vi "XML to Variable Cluster.vi"(10 "Name.Sub":string[](array[string]), 11 "After Var Name":string[](array[string])) -> (3 "Variable Clusters out":T1)   [LabVIEW 2015]
uses:
  Variable cluster.ctl
panel:
  out "Array":string[](array[string])
  out "error IO":errorcluster
  in  "error in":errorcluster
  out "Numeric":i32
  in  "Variable Clusters":T1
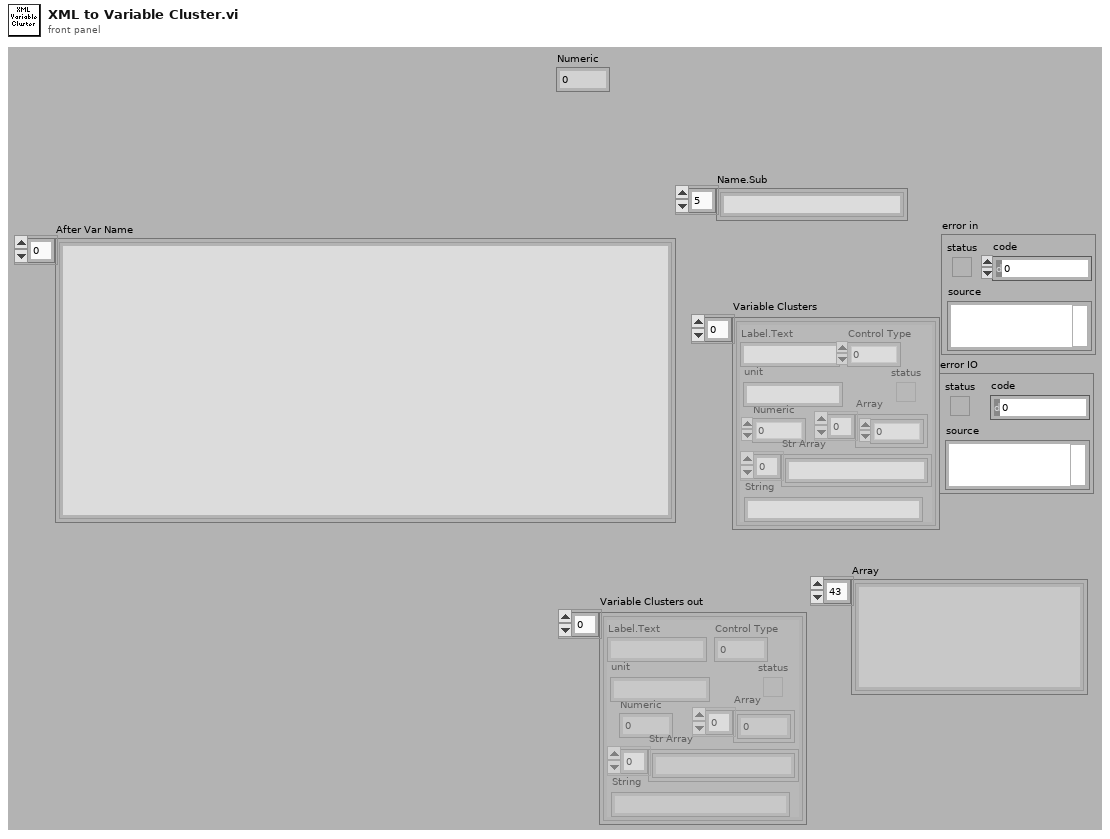
[diagram p1: front panel]
types:
  T1 = typedef "Variable cluster.ctl" = cluster{"Label.Text":string, "Control Type":u32, "Numeric":dbl, "Array":dbl[], "status":bool, "Str Array":string[], "String":string, "unit":string}[]
  T2 = cluster{"Label.Text":string, "Control Type":u32, "Numeric":dbl, "Array":dbl[], "status":bool, "Str Array":string[], "String":string, "unit":string}
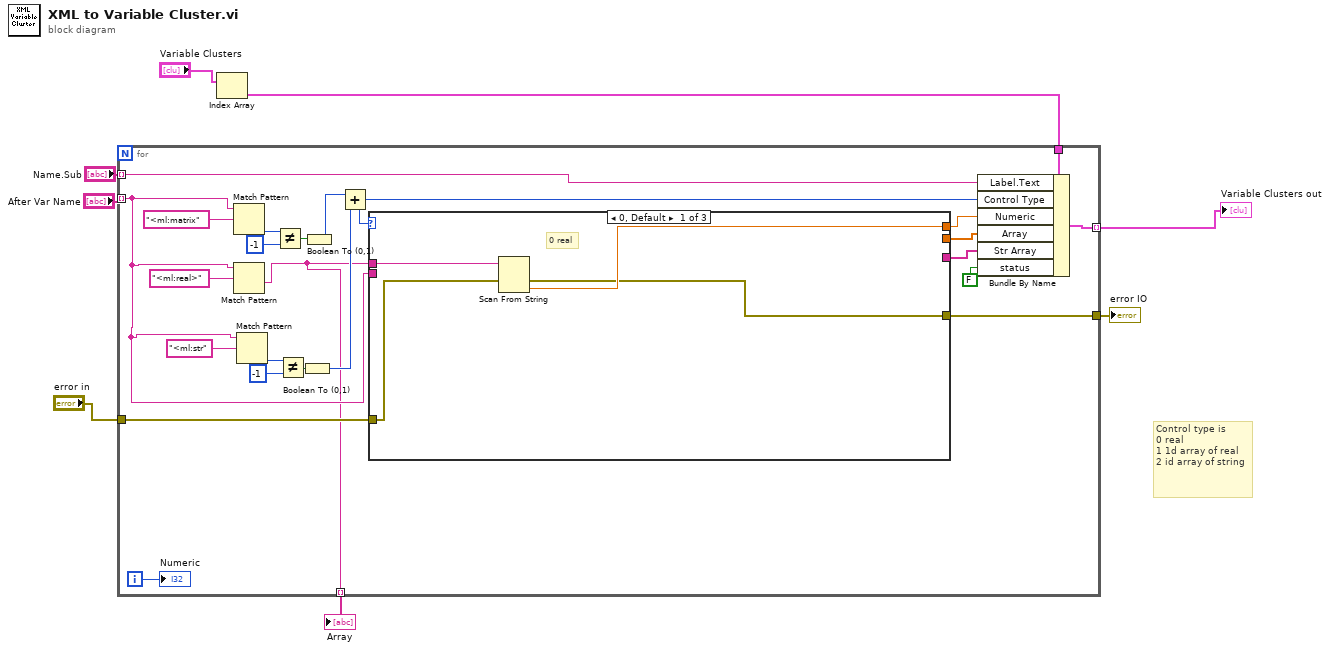
[diagram p0: block diagram]
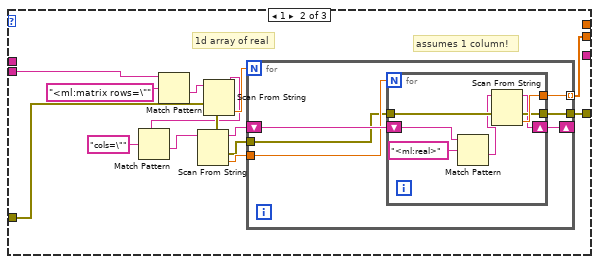
[diagram p2: hidden frame]
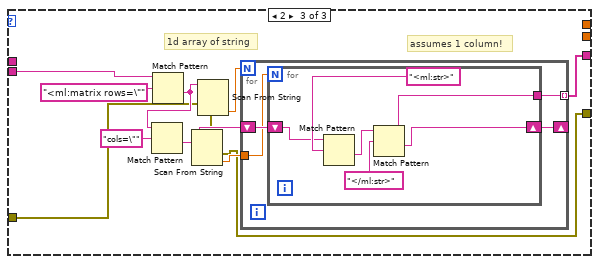
[diagram p3: hidden frame]
diagram:
  # "Control type is\n0 real\n1 1d array of real\n2 id array of string"
  n1 = Index Array(array="Variable Clusters") -> (element=w5:T2)  [unwired: 1 in]
  n2 = for {
    tunnel: "After Var Name" -> [w17] mode=indexing
    tunnel: "Name.Sub" -> [w30] mode=indexing
    tunnel: w5 -> [w32]
    tunnel: [w31] -> w4 mode=indexing
    tunnel: "error in" -> [w12]
    tunnel: [w11] -> w2
    tunnel: [w10] -> w1 mode=indexing
    i -> [w13]
    n3 = Match Pattern(string=w17, regular expression="<ml:matrix") -> (offset past match=w28:i32)  [unwired: 1 in, 3 out]
    n4 = Match Pattern(string=w17, regular expression="<ml:real>") -> (after substring=w10:string)  [unwired: 1 in, 3 out]
    n5 = Match Pattern(string=w17, regular expression="<ml:str") -> (offset past match=w24:i32)  [unwired: 1 in, 3 out]
    n6 = Not Equal?(x=w28, y=-1) -> (x != y?=w22:bool)
    n7 = Not Equal?(x=w24, y=-1) -> (x != y?=w20:bool)
    n8 = Boolean To (0,1)(Boolean=w20) -> (0, 1=w19:i16)
    n9 = Boolean To (0,1)(Boolean=w22) -> (0, 1=w21:i16)
    n10 = Add(x=w21, y=w19) -> (x+y=w18:i16)
    n11 = case shown="0, Default" w18 {
      tunnel: w17 -> [_ w50 w72]
      tunnel: w10 -> [w36 _ _]
      tunnel: [w35 _ _] -> w16
      tunnel: [_ w47 _] -> w15
      tunnel: [_ _ w71] -> w14
      tunnel: w12 -> [w34 w44 w66]
      tunnel: [w33 w41 w64] -> w11
      frame 0, Default {
        # "0 real"
        n12 = Scan From String(input string=w36, error in=w34) -> (error out=w33:errorcluster, output 1=w35:dbl)  [unwired: 3 in, 2 out]
      }
      frame 1 {
        # "assumes 1 column!"
        # "1d array of real"
        n13 = Match Pattern(string=w50, regular expression="<ml:matrix rows=\"") -> (after substring=w40:string)  [unwired: 1 in, 3 out]
        n14 = Scan From String(input string=w40, error in=w44) -> (remaining string=w39:string, error out=w43:errorcluster, output 1=w45:dbl)  [unwired: 3 in, 1 out]
        n15 = Match Pattern(string=w39, regular expression="cols=\"") -> (after substring=w38:string)  [unwired: 1 in, 3 out]
        n16 = Scan From String(input string=w38, error in=w43) -> (remaining string=w37:string, error out=w42:errorcluster, output 1=w46:dbl)  [unwired: 3 in, 1 out]
        n17 = for {
          N: w45 -> [_]
          shift-right: [w56] -> _
          shift-left: w37 -> [w55]
          tunnel: w46 -> [w54]
          tunnel: [w53] -> w47 mode=indexing
          tunnel: w42 -> [w52]
          tunnel: [w51] -> w41
          n18 = for {
            N: w54 -> [_]
            shift-right: [w58] -> w56
            shift-left: w55 -> [w62]
            tunnel: [w61] -> w53
            tunnel: w52 -> [w60]
            tunnel: [w59] -> w51
            n19 = Match Pattern(string=w62, regular expression="<ml:real>") -> (after substring=w57:string)  [unwired: 1 in, 3 out]
            n20 = Scan From String(input string=w57, error in=w60) -> (remaining string=w58:string, error out=w59:errorcluster, output 1=w61:dbl)  [unwired: 3 in, 1 out]
          }
        }
      }
      frame 2 {
        # "assumes 1 column!"
        # "1d array of string"
        n21 = Match Pattern(string=w72, regular expression="<ml:matrix rows=\"") -> (after substring=w68:string)  [unwired: 1 in, 3 out]
        n22 = Match Pattern(string=w68, regular expression="cols=\"") -> (after substring=w67:string)  [unwired: 1 in, 3 out]
        n23 = Scan From String(input string=w68, error in=w66) -> (error out=w65:errorcluster, output 1=w70:dbl)  [unwired: 3 in, 2 out]
        n24 = Scan From String(input string=w67, error in=w65) -> (error out=w64:errorcluster, output 1=w69:dbl)  [unwired: 3 in, 2 out]
        n25 = for {
          N: w70 -> [_]
          shift-right: [w78] -> _
          shift-left: w67 -> [w77]
          tunnel: w69 -> [w76]
          tunnel: [w75] -> w71 mode=indexing
          n26 = for {
            N: w76 -> [_]
            shift-right: [w79] -> w78
            shift-left: w77 -> [w83]
            tunnel: [w82] -> w75
            n27 = Match Pattern(string=w83, regular expression="<ml:str>") -> (after substring=w81:string)  [unwired: 1 in, 3 out]
            n28 = Match Pattern(string=w81, regular expression="</ml:str>") -> (before substring=w82:string, after substring=w79:string)  [unwired: 1 in, 2 out]
          }
        }
      }
    }
    n29 = Bundle By Name(cluster=w32, "Label.Text"=w30, "Control Type"=w18, "Numeric"=w16, "Array"=w15, "Str Array"=w14, "status"=FALSE ("x = y?")) -> (w31:T2)
    "Numeric" <- w13
  }
  "Variable Clusters out" <- w4
  "error IO" <- w2
  "Array" <- w1
